vi "Set VI.vi"(8 "error in":errorcluster, 10 "VI":refnum<vi>, 11 "Demo in":refnum<class "Demo.lvclass">) -> (0 "error out":errorcluster, 3 "Demo out":refnum<class "Demo.lvclass">)   [LabVIEW 2020, in "Demo.lvclass"]
uses:
  Demo.lvclass
  Demo.lvclass/Demo.ctl
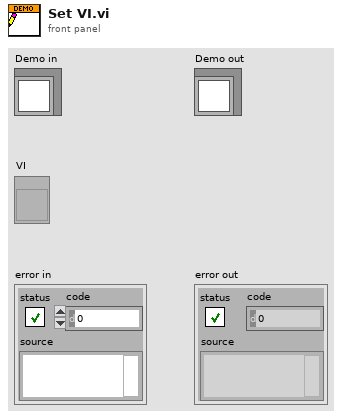
[diagram p1: front panel]
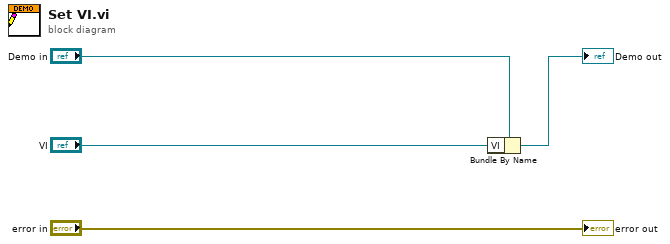
[diagram p0: block diagram]
diagram:
  n1 = Bundle By Name(cluster="Demo in", "VI"="VI") -> (→"Demo out":refnum<class "Demo.lvclass">)
  "error out" <- "error in"
